vi "Temperature Limit.vi"() -> ()   [LabVIEW 2015]
doc: "This VI simulates the acquisition of temperature, graphs the temperature, and notifies the user if the temperature is over the limit."
panel:
  in  "Start":bool
  in  "Delta t (ms)":i32(slide)=400 scale=50.0..500.0
  in  "Stop":bool
  in  "High Limit":dbl=28.0 format="%.2f"
  out "Temperature":cluster{"Temperature":dbl, "High Limit":dbl}(graph)={"Temperature"=85.88749999999999, "High Limit"=80.0}
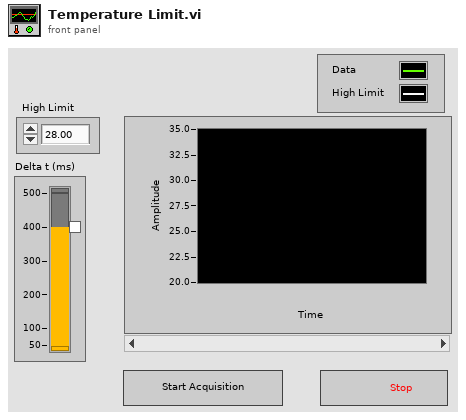
[diagram p1: front panel]
types:
  T1 = cluster{"Temperature Value":dbl, "High Limit":dbl}
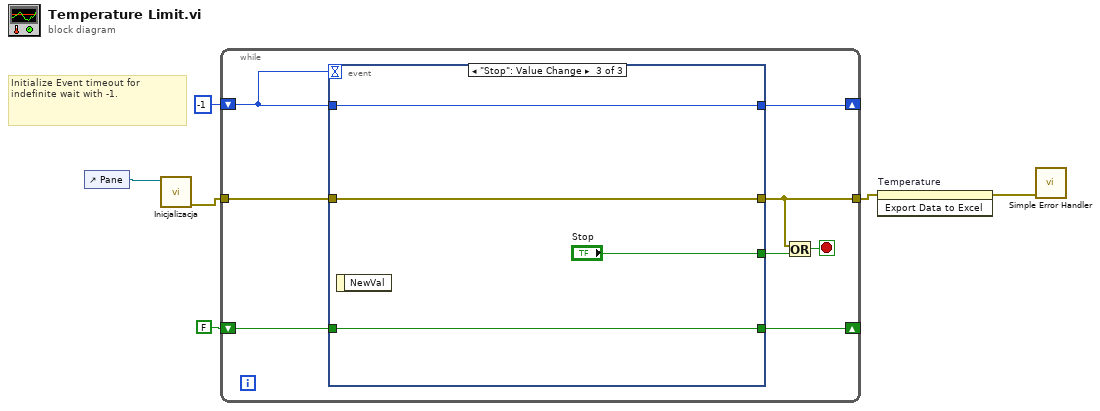
[diagram p0: block diagram]
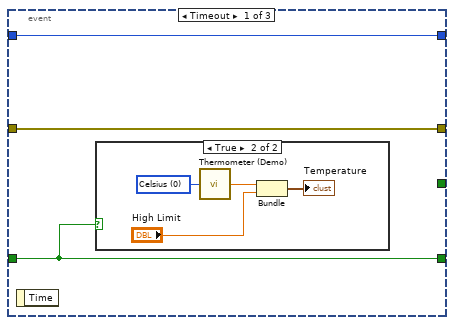
[diagram p2: hidden frame]
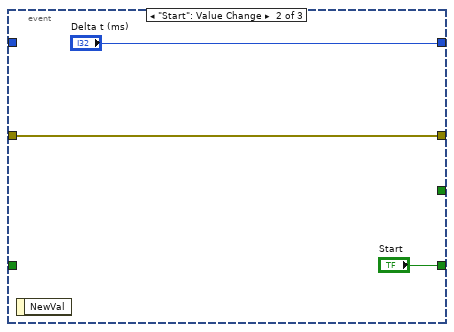
[diagram p4: hidden frame]
diagram:
  # "Initialize Event timeout for indefinite wait with -1."
  n1 = control-ref of="Pane"() -> (w1:refnum<vi>)
  n2 = call "Inicjalizacja.vi"("Pane in"=w1) -> ("error out"=w4:errorcluster)  [unwired: 10 in]
  n3 = while {
    tunnel: w4 -> [w14]
    tunnel: [w12] -> w3
    shift-right: [w10] -> _
    shift-left: FALSE ("Start") -> [w9]
    shift-right: [w8] -> _
    shift-left: -1 ("Delta t (ms)") -> [w7]
    stop <- w13 stop-if-true
    n4 = event shown="[2] \"Stop\": Value Change" {
      selector: _ -> [_ _ _]
      dyn-events: _ -> [_ _ _]
      timeout: w7 -> [_ _ _]
      tunnel: [_ _ "Stop"] -> w11
      tunnel: w14 -> [w17 w22 w27]
      tunnel: [w17 w22 w27] -> w12
      tunnel: [w15 "Start" w26] -> w10
      tunnel: w9 -> [w15 _ w26]
      tunnel: [w16 "Delta t (ms)" w25] -> w8
      tunnel: w7 -> [w16 _ w25]
      event Timeout {
        n5 = event-data() -> ()  [unwired: 1 in, 1 out]
        n6 = case shown="True" w15 {
          frame False {
          }
          frame True {
            w18 = u16 0 items=["Celsius", "Fahrenheit"] ("Units (0: Celsius)")
            n7 = call "Thermometer (Demo).vi"("Units (0: Celsius)"=w18) -> ("Temperature Value"=w19:dbl)
            n8 = Bundle("Temperature Value"=w19, "High Limit"="High Limit") -> (→"Temperature":T1)  [unwired: 1 in]
          }
        }
      }
      event "Start": Value Change {
        n9 = event-data() -> ()  [unwired: 1 in, 1 out]
      }
      event "Stop": Value Change {
        n10 = event-data() -> ()  [unwired: 1 in, 1 out]
      }
    }
    n11 = Or(x=w12, y=w11) -> (x .or. y?=w13:bool)
  }
  n12 = invoke on="Temperature" class="WFChart (strict)" method="Export Data to Excel"(error in=w3) -> (error out=w2:errorcluster)  [unwired: 2 in, 2 out]
  n13 = call <vilib>:"Simple Error Handler.vi"("error in (no error)"=w2) -> ()  [unwired: 4 in, 5 out]
